vi "Read Log.vi"(8 "error in (no error)":errorcluster, 10 "Log Path":path, 11 "Layout in":refnum<class "Layout.lvclass">) -> (0 "error out":errorcluster, 2 "Log":string, 3 "Layout out":refnum<class "Layout.lvclass">)   [LabVIEW 2019, in "TSC Event Logger.lvlib" / "Layout.lvclass"]
uses:
  Layout.lvclass
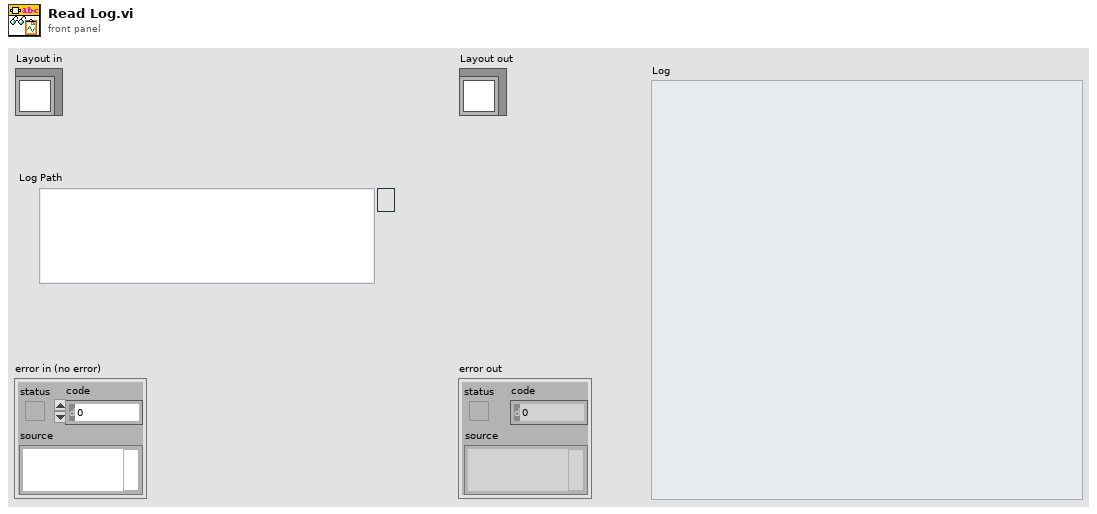
[diagram p1: front panel]
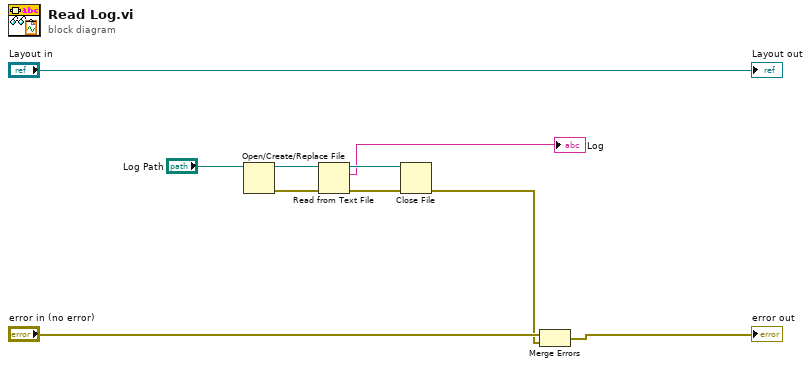
[diagram p0: block diagram]
diagram:
  n1 = Open/Create/Replace File(file path (use dialog)="Log Path") -> (refnum out=w7:refnum<file>, error out=w6:errorcluster)  [unwired: 5 in, 1 out]
  n2 = Read from Text File(file (use dialog)=w7, error in=w6) -> (refnum out=w5:refnum<file>, text=→"Log":string, error out=w4:errorcluster)  [unwired: 2 in, 1 out]
  n3 = Close File(refnum=w5, error in=w4) -> (error out=w1:errorcluster)  [unwired: 1 out]
  n4 = Merge Errors("error in (no error)", w1) -> (→"error out":errorcluster)
  "Layout out" <- "Layout in"
